vi "VI1.vi"(8 "Input":dbl=4.0) -> (0 "Output":dbl)   [LabVIEW 2023]
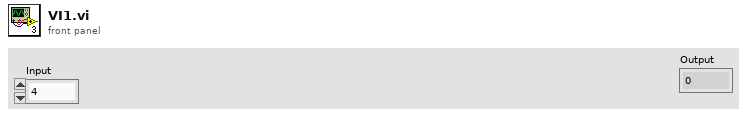
[diagram p1: front panel]
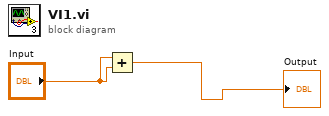
[diagram p0: block diagram]
diagram:
  n1 = Add(x="Input", y="Input") -> (x+y=→"Output":dbl)
